vi "Beam Size.vi"(11 "Best Rectangle":T1(array[cluster])) -> (2 "Y Size":dbl, 3 "X Size":dbl)   [LabVIEW 2011]
uses:
  <vilib>/Analysis/NI_AALBase.lvlib
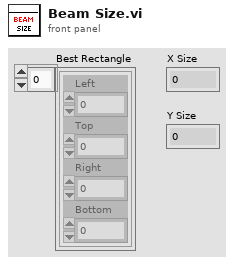
[diagram p1: front panel]
types:
  T1 = cluster{"Left":dbl, "Top":dbl, "Right":dbl, "Bottom":dbl}[]
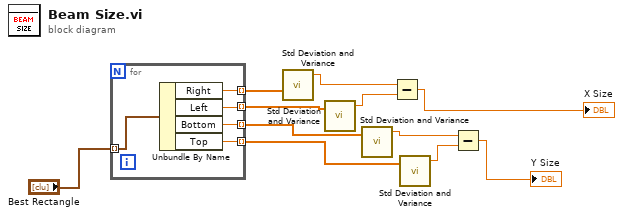
[diagram p0: block diagram]
diagram:
  n1 = for {
    tunnel: "Best Rectangle" -> [w16] mode=indexing
    tunnel: [w15] -> w2 mode=indexing
    tunnel: [w14] -> w3 mode=indexing
    tunnel: [w13] -> w4 mode=indexing
    tunnel: [w12] -> w5 mode=indexing
    n2 = Unbundle By Name(w16) -> ("Right"=w15:dbl, "Left"=w14:dbl, "Bottom"=w13:dbl, "Top"=w12:dbl)
  }
  n3 = call <vilib>:"Std Deviation and Variance.vi"("X"=w2) -> ("mean"=w6:dbl)  [unwired: 1 in, 2 out]
  n4 = call <vilib>:"Std Deviation and Variance.vi"("X"=w3) -> ("mean"=w7:dbl)  [unwired: 1 in, 2 out]
  n5 = call <vilib>:"Std Deviation and Variance.vi"("X"=w4) -> ("mean"=w8:dbl)  [unwired: 1 in, 2 out]
  n6 = Subtract(x=w6, y=w7) -> (x-y=→"X Size":dbl)
  n7 = call <vilib>:"Std Deviation and Variance.vi"("X"=w5) -> ("mean"=w9:dbl)  [unwired: 1 in, 2 out]
  n8 = Subtract(x=w8, y=w9) -> (x-y=→"Y Size":dbl)
